vi "Kaelus PFE Set Stimulus.vi"(7 "Kaelus PFE":T2, 8 "error in (no error)":errorcluster, 10 "PFE Position":T1, 11 "DAQmx Dev Name (FEModule)":string) -> (0 "error out":errorcluster, 3 "DAQmx Dev Name (FEModule)":string)   [LabVIEW 2011]
uses:
  TypeDefs/Kaelus PFE Instrument Info.ctl
  BPIMCore EXT/HW IO/PIM Parameters.ctl
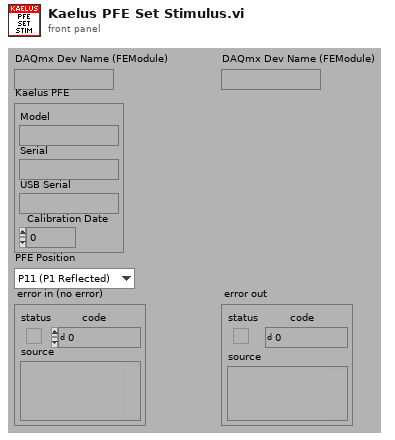
[diagram p1: front panel]
types:
  T1 = typedef "PIM Parameters.ctl" = enum16{"P11 (P1 Reflected)", "P12 (P2 Through)", "P21 (P1 Through)", "P22 (P2 Reflected)"}
  T2 = typedef "Kaelus PFE Instrument Info.ctl" = cluster{"Model":string, "Serial":string, "USB Serial":string, "Calibration Date":dbl}
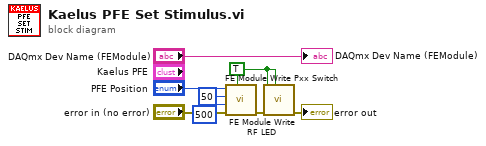
[diagram p0: block diagram]
diagram:
  w3 = TRUE
  n1 = call "FE Module Write Pxx Switch.vi"("Hardware Present (f)"=w3, "error in (no error)"="error in (no error)", "CAP Recharge time (100ms)"=u32 500, "Switch pulse length (35ms)"=u32 50, "P-Parameter"="PFE Position") -> ("error out"=w5:errorcluster)  [unwired: 3 in]
  n2 = call "FE Module Write RF LED.vi"("Hardware Present (f)"=w3, "error in (no error)"=w5, "ON? (F: OFF)"=w3) -> ("error out"=→"error out":errorcluster)  [unwired: 5 in]
  "DAQmx Dev Name (FEModule)" <- "DAQmx Dev Name (FEModule)"
